vi "Read Value Bit Width.vi"(8 "error in (no error)":errorcluster, 11 "NT Scalar (Numeric) in":refnum<class "NT Scalar (Numeric).lvclass">) -> (0 "error out":errorcluster, 2 "value bit width":i32, 3 "NT Scalar (Numeric) out":refnum<class "NT Scalar (Numeric).lvclass">)   [LabVIEW 2020, in "PV Access.lvlib" / "PV Data.lvlib" / "NT Scalar (Numeric).lvclass"]
uses:
  NT Scalar (Numeric).lvclass
  NT Scalar (Numeric).lvclass/NT Scalar (Numeric).ctl
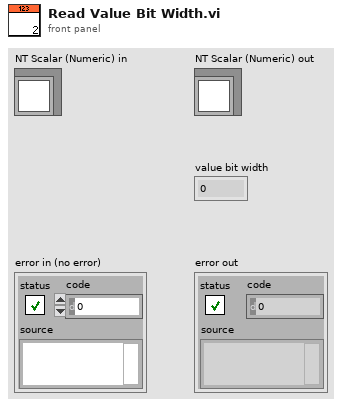
[diagram p1: front panel]
types:
  T1 = typedef "PV Access.lvlib/PV Data.lvlib/Type Code.ctl" = enum8{"Null", "Bool", "BoolA", "Int8", "Int8A", "Int16", "Int16A", "Int32", "Int32A", "Int64", "Int64A", "UInt8", "UInt8A", "UInt16", "UInt16A", "UInt32", "UInt32A", "UInt64", "UInt64A", "Float32", "Float32A", "Float64", "Float64A", "String", "StringA", "Struct", "StructA", "Union", "UnionA", "Any", "AnyA"}
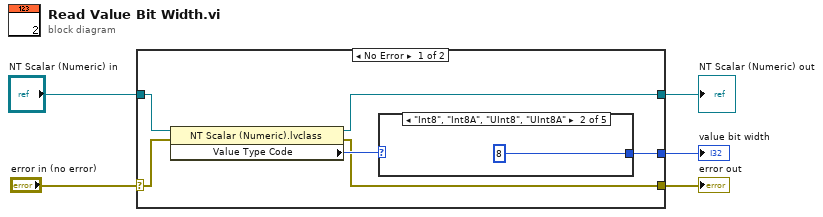
[diagram p0: block diagram]
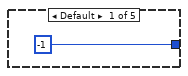
[diagram p2: hidden frame]
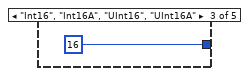
[diagram p3: hidden frame]
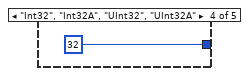
[diagram p4: hidden frame]
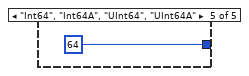
[diagram p5: hidden frame]
diagram:
  n1 = case shown="No Error" "error in (no error)" {
    selector: "error in (no error)" -> [w8 w18]
    tunnel: [w7 w18] -> w4
    tunnel: [w10 w17] -> w2
    tunnel: "NT Scalar (Numeric) in" -> [w11 w17]
    tunnel: [w6 _] -> w1
    frame No Error {
      n2 = property class="NT Scalar (Numeric).lvclass"(reference=w11, error in=w8) -> (reference out=w10:refnum<class "NT Scalar (Numeric).lvclass">, error out=w7:errorcluster, "Value Type Code"=w9:T1)
      n3 = case shown="\"Int8\", \"Int8A\", \"UInt8\", \"UInt8A\"" w9 {
        tunnel: [-1 8 16 32 64] -> w6
        frame Default {
        }
        frame "Int8", "Int8A", "UInt8", "UInt8A" {
        }
        frame "Int16", "Int16A", "UInt16", "UInt16A" {
        }
        frame "Int32", "Int32A", "UInt32", "UInt32A" {
        }
        frame "Int64", "Int64A", "UInt64", "UInt64A" {
        }
      }
    }
    frame Error {
    }
  }
  "error out" <- w4
  "NT Scalar (Numeric) out" <- w2
  "value bit width" <- w1
